vi "Cannon Process.vi"   [LabVIEW 2013]
uses:
  Cannon Global.vi
types:
  T1 = typedef "WPI_RelayValue.ctl" = enum16{"Off", "On", "Forward", "Reverse"}
  T2 = cluster{"Angle":dbl, "Clutch MS":bool, "Ball MS":bool, "Motor VBus":dbl, "Clutch ":T1, "LeFireatwill":bool, "Arm":bool, "Armed":bool, "Fire!":bool}
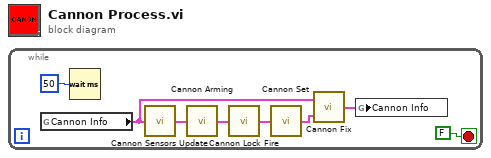
[diagram p0: block diagram]
diagram:
  n1 = while {
    stop <- FALSE stop-if-true
    n2 = global read "Cannon Global.vi" "Cannon Info"() -> (w3:T2)
    n3 = Wait (ms)(milliseconds to wait=u32 50) -> ()  [unwired: 1 out]
    n4 = call "Cannon Sensors Update.vi"("Cannon Info In"=w3) -> ("Cannon Info Out"=w7:T2)
    n5 = call "Cannon Arming.vi"("Cannon Info In"=w7) -> ("Cannon Info Out"=w6:T2)
    n6 = call "Cannon Lock Fire.vi"("Cannon Info In"=w6) -> ("Cannon Info Out"=w5:T2)
    n7 = call "Cannon Set.vi"("Cannon Info In"=w5) -> ("Cannon Info Out"=w4:T2)
    n8 = call "Cannon Fix.vi"("Cannon Info Modified"=w4, "Cannon Info Original"=w3) -> ("Cannon Info Fixed"=w2:T2)
    n9 = global write "Cannon Global.vi" "Cannon Info"(w2) -> ()
  }
